vi "GlobalDataSelectArray.vi"() -> ()   [LabVIEW 2013]
panel:
  out "Data Select Array":bool[](array[boolean])
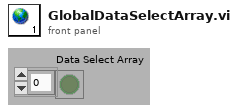
[diagram p1: front panel]
diagram:
